vi "absCalcPlot.vi"(5 "file path (dialog if empty)":path, 6 "Cell Calibration, mV/mW":dbl=600000.0, 7 "save?":bool, 8 "Error In":errorcluster, 9 "PD Values":cluster{dbl, dbl, dbl, dbl}, 10 "bkg values":cluster{dbl, dbl, dbl, dbl}, 11 "Mic Values":cluster{dbl, dbl, dbl, dbl}) -> (0 "Error Out":errorcluster, 1 "aae":dbl, 2 "Time Series":cluster{dbl, dbl, dbl, dbl}, 3 "Spectrum":cluster{dbl[], "Best Power Fit":dbl[]}[](graph))   [LabVIEW 2011]
uses:
  <vilib>/Analysis/NI_AALPro.lvlib
panel:
  out "output cluster":cluster{i32[], "Best Power Fit":dbl[]}
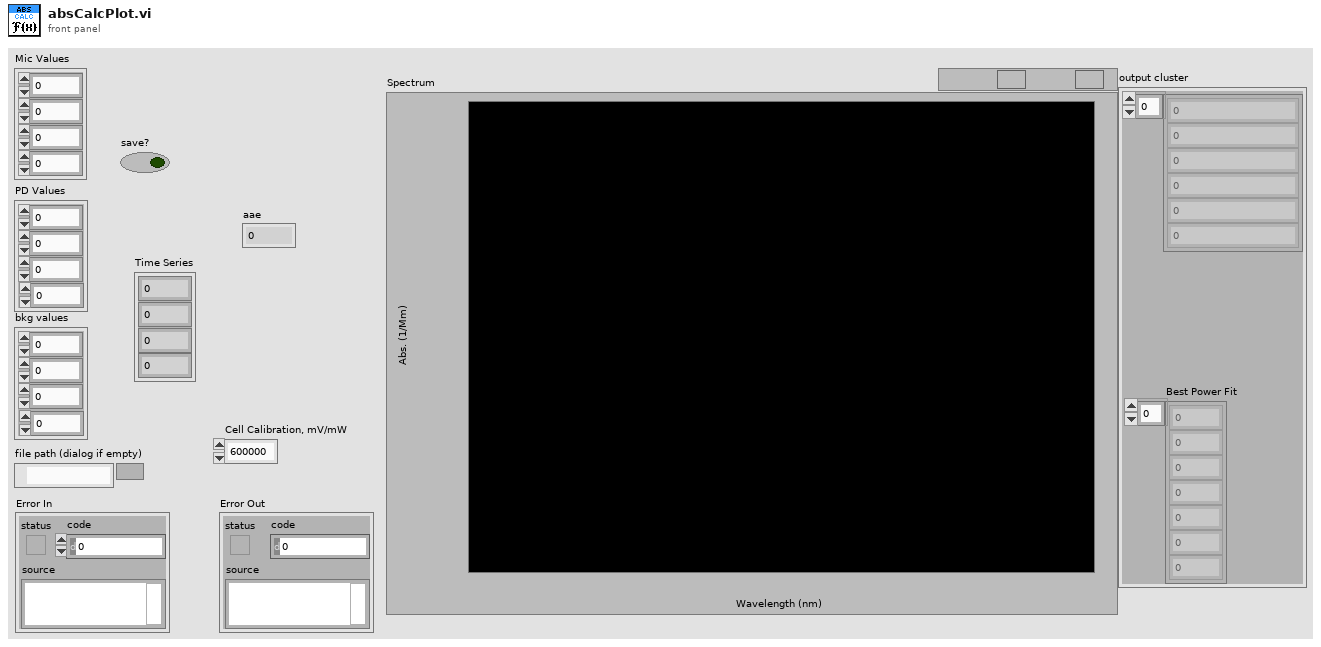
[diagram p1: front panel]
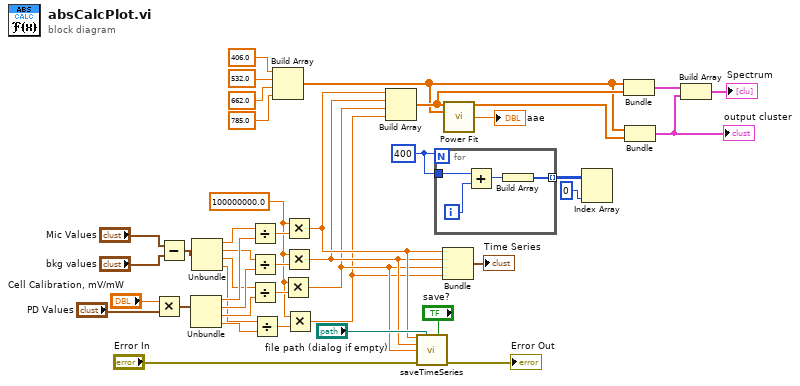
[diagram p0: block diagram]
diagram:
  w3 = 100000000.0 ("element")
  w22 = 400
  n1 = Multiply(x="Cell Calibration, mV/mW", y="PD Values") -> (x*y=w36:cluster{dbl, dbl, dbl, dbl})
  n2 = Subtract(x="Mic Values", y="bkg values") -> (x-y=w24:cluster{dbl, dbl, dbl, dbl})
  n3 = Unbundle(w36) -> (w37:dbl, w38:dbl, w39:dbl, w4:dbl)
  n4 = Unbundle(w24) -> (w31:dbl, w32:dbl, w33:dbl, w5:dbl)
  n5 = Divide(x=w31, y=w37) -> (x/y=w16:dbl)
  n6 = Divide(x=w32, y=w38) -> (x/y=w15:dbl)
  n7 = Divide(x=w33, y=w39) -> (x/y=w14:dbl)
  n8 = Divide(x=w5, y=w4) -> (x/y=w6:dbl)
  n9 = Build Array(406.0 ("element"), 532.0 ("element"), 662.0 ("element"), 785.0 ("element")) -> (w11:dbl[])
  n10 = Multiply(x=w3, y=w14) -> (x*y=w7:dbl)
  n11 = Multiply(x=w3, y=w16) -> (x*y=w9:dbl)
  n12 = Multiply(x=w3, y=w15) -> (x*y=w8:dbl)
  n13 = Multiply(x=w3, y=w6) -> (x*y=w1:dbl)
  n14 = Build Array(w9, w8, w7, w1) -> (w12:dbl[])
  n15 = call "saveTimeSeries.vi"("405nm"=w9, "file path (dialog if empty)"="file path (dialog if empty)", "save?"="save?", "532nm"=w8, "660nm"=w7, "Error In"="Error In") -> ("Error Out"=→"Error Out":errorcluster)  [unwired: 9 in]
  n16 = for {
    N: w22 -> [_]
    tunnel: w22 -> [w45]
    tunnel: [w43] -> w20 mode=indexing
    i -> [w46]
    n17 = Add(x=w45, y=w46) -> (x+y=w44:i32)
    n18 = Build Array(w44) -> (w43:i32[])
  }
  n19 = Bundle(w9, w8, w7, w1) -> (→"Time Series":cluster{dbl, dbl, dbl, dbl})  [unwired: 1 in]
  n20 = call <vilib>:"Power Fit.vi"("Y"=w12, "X"=w11) -> ("Best Power Fit"=w21:dbl[], "power"=→"aae":dbl)  [unwired: 8 in, 4 out]
  n21 = Index Array(array=w20, index (col)=0 ("index (row)")) -> ()  [unwired: 1 in, 1 out]
  n22 = Bundle(w11, w12) -> (w10:cluster{dbl[], dbl[]})  [unwired: 1 in]
  n23 = Bundle(w11, "Best Power Fit"=w21) -> (w19:cluster{dbl[], "Best Power Fit":dbl[]})  [unwired: 1 in]
  "output cluster" <- w19
  n24 = Build Array(w10, w19) -> (→"Spectrum":cluster{dbl[], "Best Power Fit":dbl[]}[])
